vi "Q_32B_v2.vi"(11 "Q_32B":dbl) -> (0 "LL":u8, 1 "HL":u8, 2 "LH":u8, 3 "HH":u8)   [LabVIEW 2017]
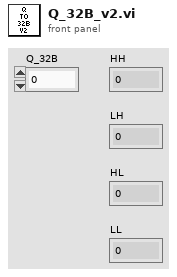
[diagram p1: front panel]
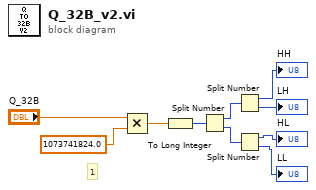
[diagram p0: block diagram]
diagram:
  # "1"
  n1 = Multiply(x="Q_32B", y=1073741824.0) -> (x*y=w1:dbl)
  n2 = To Long Integer(number=w1) -> (32bit integer=w6:i32)
  n3 = Split Number(x=w6) -> (hi(x)=w4:u16, lo(x)=w5:u16)
  n4 = Split Number(x=w4) -> (hi(x)=→"HH":u8, lo(x)=→"LH":u8)
  n5 = Split Number(x=w5) -> (hi(x)=→"HL":u8, lo(x)=→"LL":u8)
